vi "UTF16 Encoding to UTF8 Encoding.vi"(6 "Big Endian?":bool, 8 "error in (no error)":errorcluster, 9 "UTF-16 String":string="…\u000b") -> (0 "error out":errorcluster, 1 "UTF-8 String":string)   [LabVIEW 2011]
doc: "Converts the UTF-16LE Encoded string to UTF-8 encoded string."
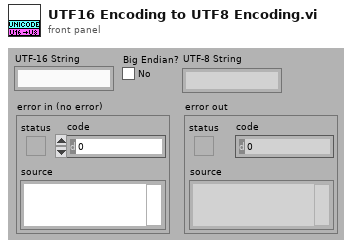
[diagram p1: front panel]
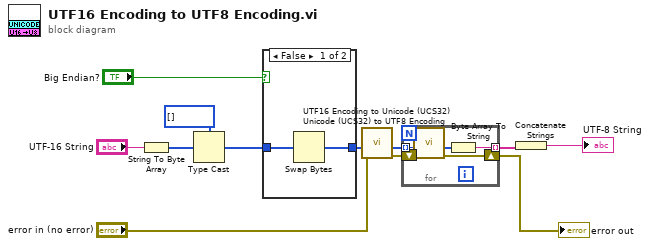
[diagram p0: block diagram]
diagram:
  n1 = String To Byte Array(string="UTF-16 String") -> (unsigned byte array=w7:u8[])
  n2 = Type Cast(type=u16[] [] ("[UTF-16]"), x=w7) -> (*(type *) &x=w8:u16[])
  n3 = case shown="False" "Big Endian?" {
    tunnel: w8 -> [w14 w15]
    tunnel: [w13 w15] -> w5
    frame False {
      n4 = Swap Bytes(anything=w14) -> (byte swapped=w13:u16[])
    }
    frame True {
    }
  }
  n5 = call "UTF16 Encoding to Unicode (UCS32).vi"("error in"="error in (no error)", "[UTF-16]"=w5) -> ("error out"=w2:errorcluster, "[UCS 32]"=w4:u32[])  [unwired: 8 in]
  n6 = for {
    tunnel: [w20] -> w12 mode=indexing
    tunnel: w4 -> [w19] mode=indexing
    shift-right: [w16] -> w1
    shift-left: w2 -> [w17]
    n7 = call "Unicode (UCS32) to UTF8 Encoding.vi"("error in (no error)"=w17, "UCS 32"=w19) -> ("error out"=w16:errorcluster, "[UTF-8]"=w18:u8[])  [unwired: 8 in]
    n8 = Byte Array To String(unsigned byte array=w18) -> (string=w20:string)
  }
  "error out" <- w1
  n9 = Concatenate Strings(w12) -> (→"UTF-8 String":string)
